vi "IMAQ FPGA Data Valid Bool Array to Int x32.vi"(11 "DV In":bool[](array[boolean])=[FALSE, FALSE, FALSE, FALSE, FALSE, FALSE, FALSE, FALSE, FALSE, FALSE, FALSE, FALSE, FALSE, FALSE, FALSE, FALSE, FALSE, FALSE, FALSE, FALSE, FALSE, FALSE, FALSE, FALSE, FALSE, FALSE, FALSE, FALSE, FALSE, FALSE, FALSE, FALSE]) -> (3 "Sum DV Out":u8)   [LabVIEW 2020, in "NI_VDM_FPGA_Basics.lvlib"]
uses:
  <vilib>/visionFPGA/NI_VDM_FPGA_Basics.lvlib
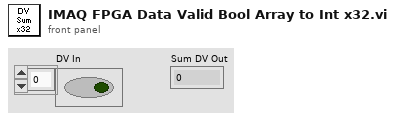
[diagram p1: front panel]
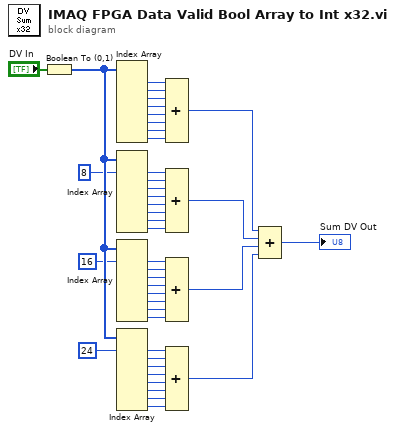
[diagram p0: block diagram]
diagram:
  n1 = Boolean To (0,1)(Boolean="DV In") -> (0, 1=w9:i16[])
  n2 = Index Array(array=w9) -> (element #1=w41:i16, element #2=w40:i16, element #3=w34:i16, element #4=w35:i16, element #5=w36:i16, element #6=w37:i16, element #7=w38:i16, element #8=w39:i16)  [unwired: 8 in]
  n3 = Index Array(array=w9, index #1=8 ("index")) -> (element #1=w26:i16, element #2=w27:i16, element #3=w33:i16, element #4=w32:i16, element #5=w31:i16, element #6=w30:i16, element #7=w29:i16, element #8=w28:i16)  [unwired: 7 in]
  n4 = Index Array(array=w9, index #1=16 ("index")) -> (element #1=w25:i16, element #2=w24:i16, element #3=w18:i16, element #4=w19:i16, element #5=w20:i16, element #6=w21:i16, element #7=w22:i16, element #8=w23:i16)  [unwired: 7 in]
  n5 = Index Array(array=w9, index #1=24 ("index")) -> (element #1=w10:i16, element #2=w11:i16, element #3=w17:i16, element #4=w16:i16, element #5=w15:i16, element #6=w14:i16, element #7=w13:i16, element #8=w12:i16)  [unwired: 7 in]
  n6 = Compound Arithmetic op=ADD(w41, w40, w34, w35, w36, w37, w38, w39) -> (w5:i16)
  n7 = Compound Arithmetic op=ADD(w26, w27, w33, w32, w31, w30, w29, w28) -> (w4:i16)
  n8 = Compound Arithmetic op=ADD(w25, w24, w18, w19, w20, w21, w22, w23) -> (w3:i16)
  n9 = Compound Arithmetic op=ADD(w10, w11, w17, w16, w15, w14, w13, w12) -> (w2:i16)
  n10 = Compound Arithmetic op=ADD(w5, w4, w3, w2) -> (→"Sum DV Out":i16)
